vi "SeverNanonisSSL.vi"() -> ()   [LabVIEW 2014]
uses:
  <userlib>/SSL Library/Controls/SSL_Data.ctl
  <userlib>/SSL Library/Controls/Ref.ctl
  <userlib>/SSL Library/SSL Lib.lvlib
panel:
  out "Auth Status":T1(ring)
  in  "User":cluster{"pass":string, "User":string}={"pass"="password", "User"="password"}
  out "User auth":bool
  out "Listener Ref":refnum<k24>
  out "Client Connected ?":bool
  in  "Ssl Protocols Type":i32(ring)=240 items=["None"=0, "Ssl2"=12, "Ssl3"=48, "Tls"=192, "Default"=240]
  in  "Client Certificate Required":bool
  in  "Input Message":string="keep alive,30000;" caption="Type Message to send"
  out "Message log":string
  in  "Port Number":i32=4001
  out "Status":string="Waiting For Client ..."
  in  "Stop Button":bool=TRUE
  in  "Restart":bool
  in  "Read":bool
  in  "Write":bool
  out "Error Out":errorcluster
  in  "Password":string="password"
  in  "Certificate Path":string="C:\\Program Files (x86)\\National Instruments\\LabVIEW 2014\\user.lib\\SSL Library\\Server.pfx"
  in  "Error In":errorcluster
  # "TCP Server over SSL"
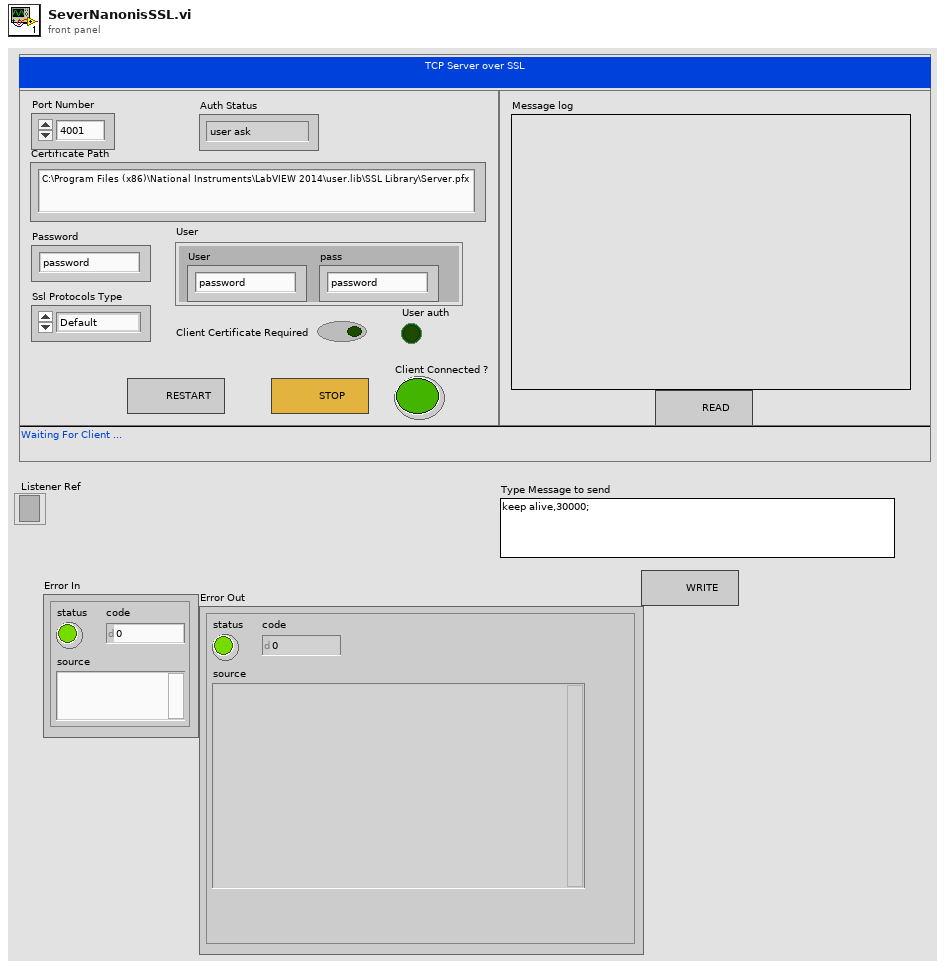
[diagram p1: front panel]
types:
  T1 = enum16{"user ask", "user", "pass ask", "pass", "auth"}
  T2 = typedef "SSL_Data.ctl" = cluster{"Listener Ref":refnum<k24>, "Certificate":refnum<k24>, "AcceptTcpClient":refnum<k24>, "SSL Stream":refnum<k24>, "Message Read":string}
  T3 = enum16{"Poll", "Open Listener", "Generate Certificate", "Wait for Client", "Open SSL Steram", "Read from SSL Stream", "Write Data to SSL Steram", "Close Connection"}
  T4 = typedef "Ref.ctl" = enum16{"Update Ref", "Read Ref", "Close Ref"}
  T5 = cluster{"Certificate Ref":refnum<k24>, "Client Certificate Required":bool, "Ssl Protocols Type":i32, "Check Certificate Revocation":bool}
  T6 = enum16{"Poll", "Open Listener", "Generate Certificate", "Wait for Client", "Open SSL Steram", "Read from SSL Stream", "Write Data to SSL Steram", "Close Connection", "Ask Username", "Ask Password", "Parse"}
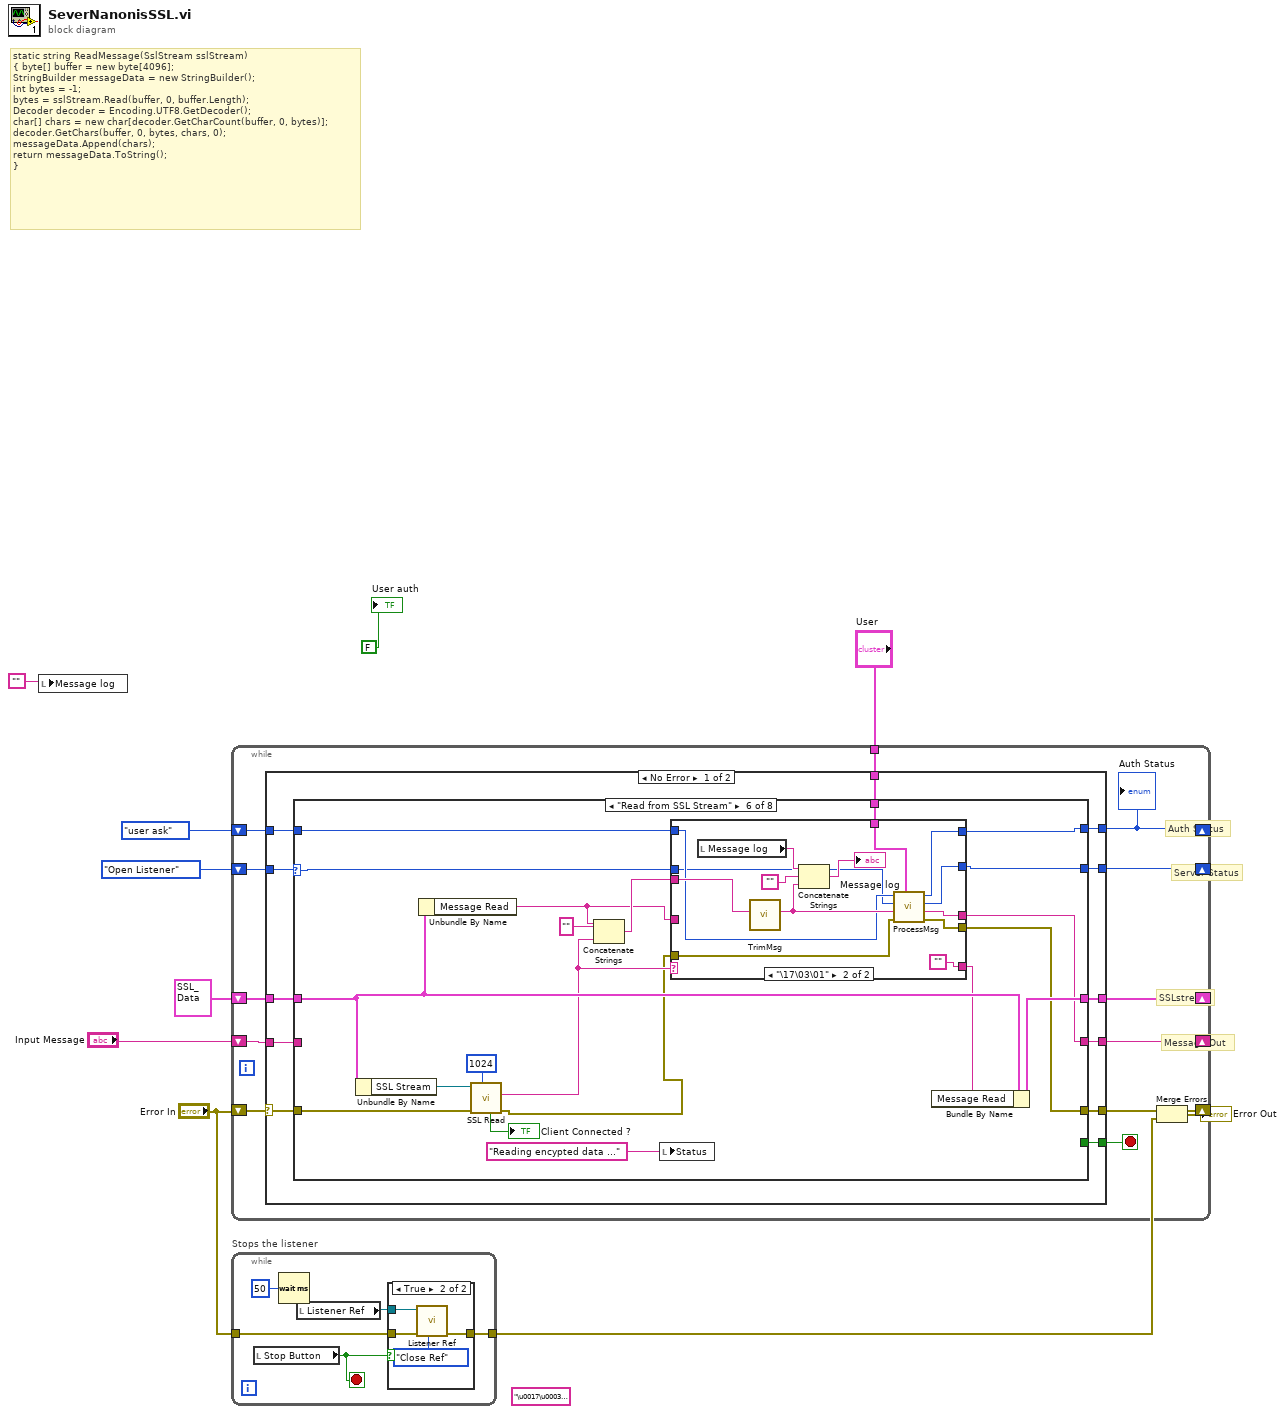
[diagram p0: block diagram]
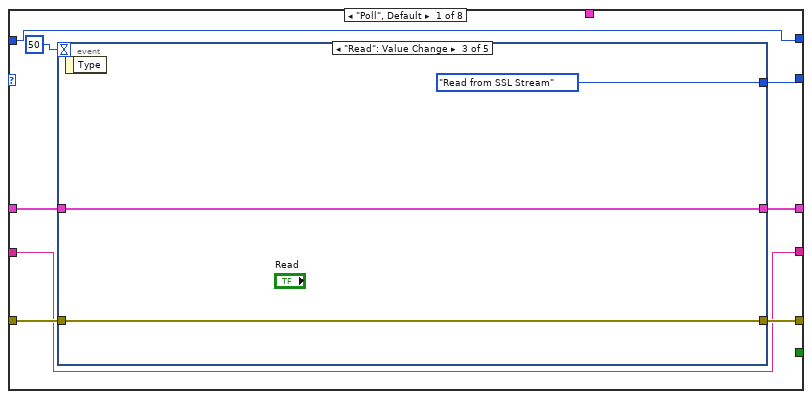
[diagram p3: hidden frame]
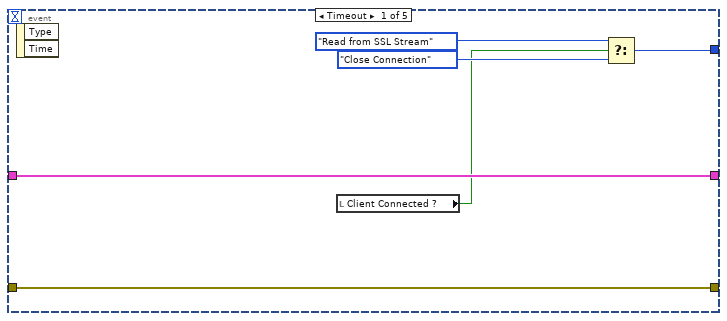
[diagram p4: hidden frame]
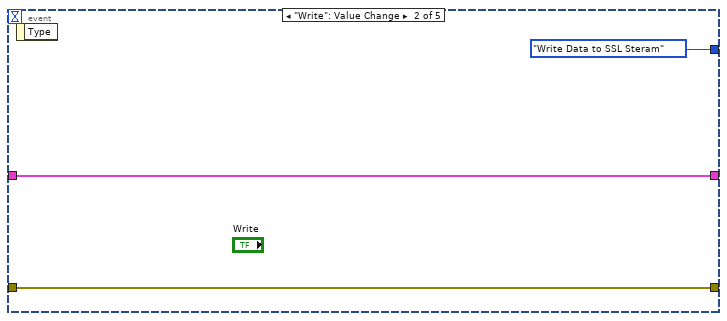
[diagram p5: hidden frame]
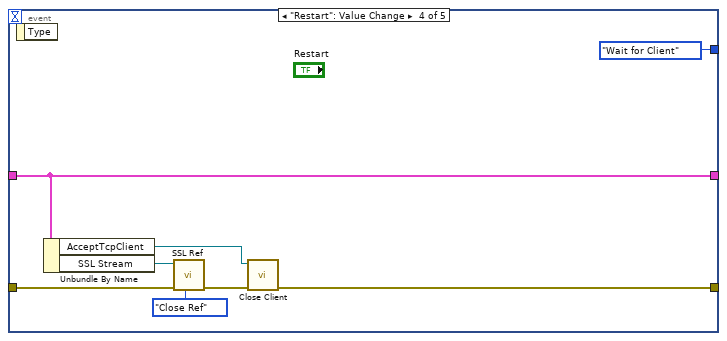
[diagram p6: hidden frame]
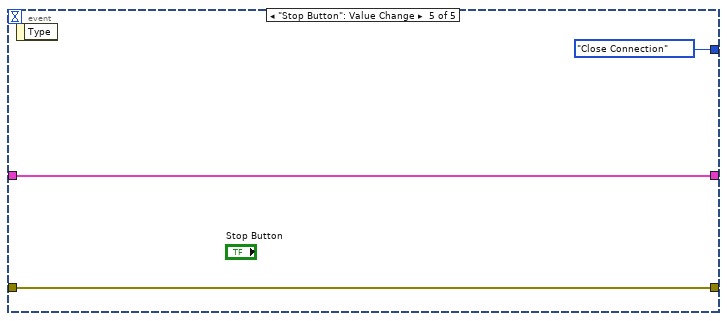
[diagram p7: hidden frame]
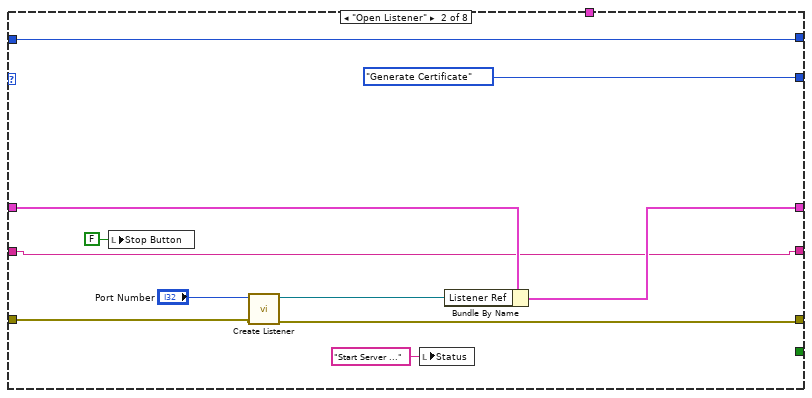
[diagram p8: hidden frame]
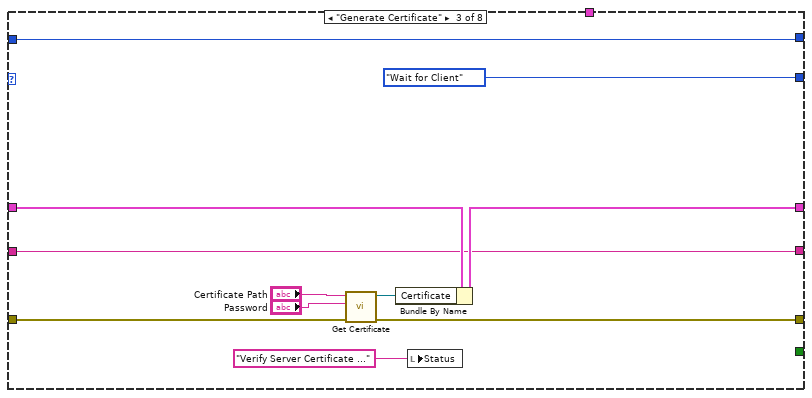
[diagram p9: hidden frame]
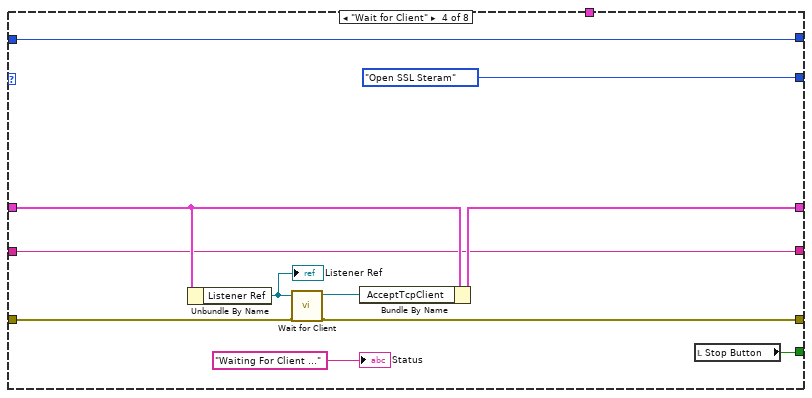
[diagram p10: hidden frame]
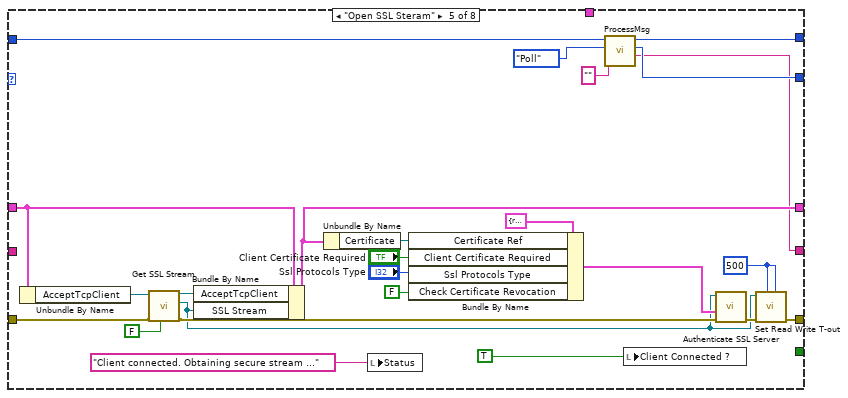
[diagram p11: hidden frame]
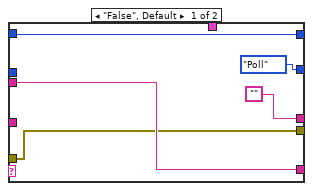
[diagram p12: hidden frame]
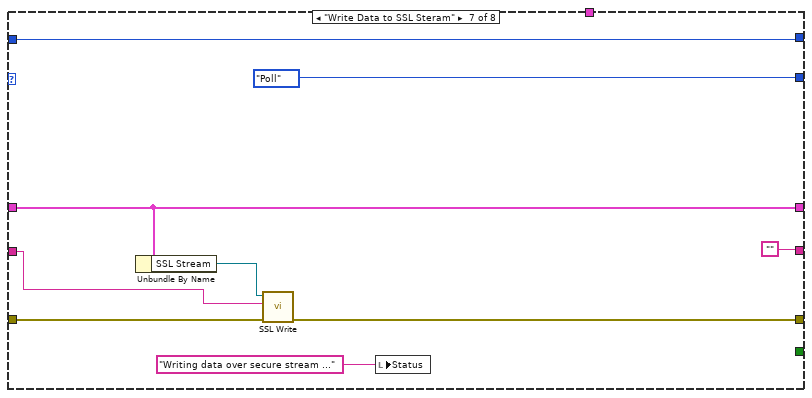
[diagram p13: hidden frame]
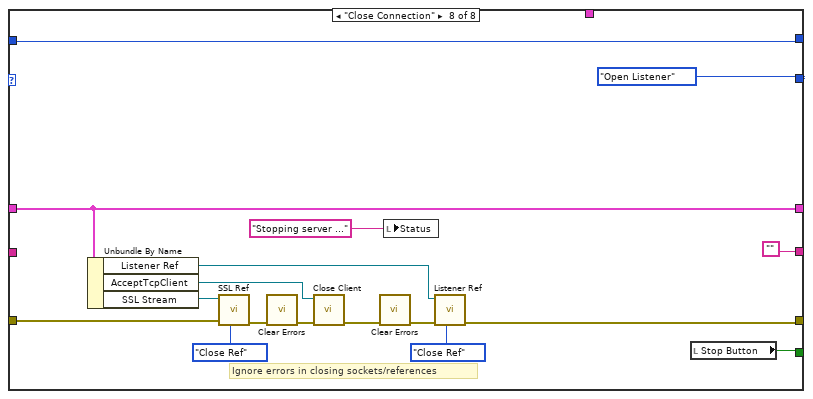
[diagram p14: hidden frame]
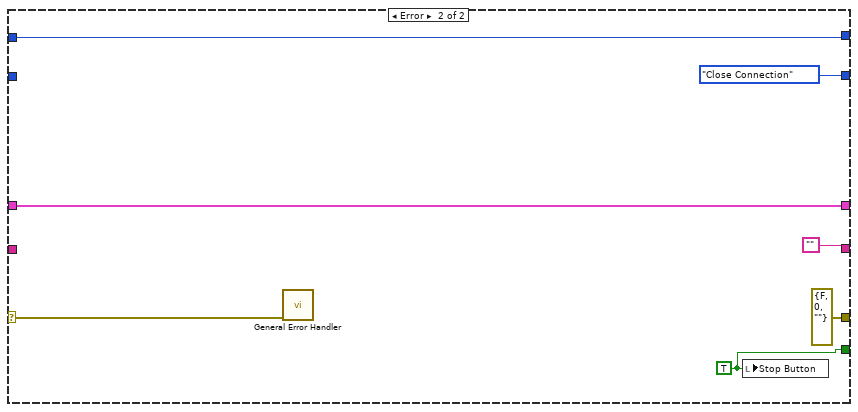
[diagram p15: hidden frame]
diagram:
  (unwired) "\u0017\u0003\u0001"
  # "Server Status"
  # "Auth Status"
  # "SSLstream"
  # "Message Out"
  # "static string ReadMessage(SslStream sslStream) \n{ byte[] buffer = new byte[4096];\nStringBuilder messageData = new StringBuilder(); \nint bytes = -1;\nbytes = sslStream.Read(buffer, 0, buffer.Length);\nDecoder decoder = Encoding.UTF8.GetDecoder(); \nchar[] chars = new char[decoder.GetCharCount(buffer, 0, bytes)]; \ndecoder.GetChars(buffer, 0, bytes, chars, 0); \nmessageData.Append(chars);\nreturn messageData.ToString();\n}"
  n1 = local write "Message log"("") -> ()
  n2 = while {
    shift-right: [w21] -> _
    shift-left: T2 {"Listener Ref"=refnum, "Certificate"=refnum, "AcceptTcpClient"=refnum, "SSL Stream"=refnum, "Message Read"=""} -> [w22]
    shift-right: [w23] -> w8
    shift-left: "Error In" -> [w20]
    shift-right: [w18] -> _
    shift-left: T3."Open Listener" -> [w19]
    shift-right: [w15] -> _
    shift-left: T1."user ask" -> [w16]
    shift-right: [w13] -> _
    shift-left: "Input Message" -> [w14]
    tunnel: "User" -> [w12]
    stop <- w17 stop-if-true
    n3 = case shown="No Error" w20 {
      selector: w20 -> [w32 w194]
      tunnel: [w35 errorcluster {"status"=FALSE, "code"=0, "source"=""} ("Error Out")] -> w23
      tunnel: w22 -> [w34 w196]
      tunnel: [w33 w196] -> w21
      tunnel: w19 -> [w31 _]
      tunnel: [w30 T3."Close Connection"] -> w18
      tunnel: [w29 w192] -> w17
      tunnel: w16 -> [w28 w191]
      tunnel: [w27 w191] -> w15
      tunnel: w14 -> [w26 _]
      tunnel: [w25 ""] -> w13
      tunnel: w12 -> [w24 _]
      frame No Error {
        n4 = case shown="\"Read from SSL Stream\"" w31 {
          selector: w31 -> [_ _ _ _ _ w130 _ _]
          tunnel: w32 -> [w41 w76 w85 w96 w124 w144 w171 w188]
          tunnel: [w40 w75 w84 w95 w109 w126 w170 w184] -> w35
          tunnel: w34 -> [w43 w70 w88 w93 w121 w140 w168 w179]
          tunnel: [w42 w69 w87 w99 w117 w139 w168 w179] -> w33
          tunnel: [w39 T3."Generate Certificate" T3."Wait for Client" T3."Open SSL Steram" w102 w129 T3."Poll" T3."Open Listener"] -> w30
          tunnel: [_ _ _ w89 _ _ _ w173] -> w29
          tunnel: w28 -> [w37 w68 w79 w91 w105 w132 w166 w174]
          tunnel: [w37 w68 w79 w91 w104 w131 w166 w174] -> w27
          tunnel: w26 -> [w36 w67 w78 w90 _ _ w165 _]
          tunnel: [w36 w67 w78 w90 w100 w128 "" ""] -> w25
          tunnel: w24 -> [_ _ _ _ _ w125 _ _]
          frame "Poll", Default {
            n5 = event shown="[2] \"Read\": Value Change" {
              selector: _ -> [_ _ _ _ _]
              dyn-events: _ -> [_ _ _ _ _]
              timeout: 50 -> [_ _ _ _ _]
              tunnel: w43 -> [w46 w52 w55 w58 w65]
              tunnel: [w46 w52 w55 w58 w65] -> w42
              tunnel: w41 -> [w45 w51 w54 w62 w66]
              tunnel: [w45 w51 w54 w60 w66] -> w40
              tunnel: [w49 T3."Write Data to SSL Steram" T3."Read from SSL Stream" T3."Wait for Client" T3."Close Connection"] -> w39
              event Timeout {
                n6 = event-data() -> ()  [unwired: 1 in, 2 out]
                n7 = local read "Client Connected ?"() -> (w44:bool)
                n8 = Select(t=T3."Read from SSL Stream", s=w44, f=T3."Close Connection") -> (s? t:f=w49:T3)
              }
              event "Write": Value Change {
                n9 = event-data() -> ()  [unwired: 1 in, 1 out]
              }
              event "Read": Value Change {
                n10 = event-data() -> ()  [unwired: 1 in, 1 out]
              }
              event "Restart": Value Change {
                n11 = event-data() -> ()  [unwired: 1 in, 1 out]
                n12 = Unbundle By Name(w58) -> ("AcceptTcpClient"=w56:refnum<k24>, "SSL Stream"=w57:refnum<k24>)
                n13 = call <userlib>:"SSL Ref.vi"("Action"=Ref."Close Ref", "Error In"=w62, "SSL Stream"=w57) -> ("Error Out"=w61:errorcluster)  [unwired: 7 in, 1 out]
                n14 = call <userlib>:"Close Client.vi"("Error In"=w61, "Client Ref"=w56) -> ("Error Out"=w60:errorcluster)  [unwired: 9 in]
              }
              event "Stop Button": Value Change {
                n15 = event-data() -> ()  [unwired: 1 in, 1 out]
              }
            }
          }
          frame "Open Listener" {
            n16 = local write "Stop Button"(FALSE ("Stop Button")) -> ()
            n17 = call <userlib>:"Create Listener.vi"("Error In"=w76, "Port Number"="Port Number") -> ("Error Out"=w75:errorcluster, "Listener"=w71:refnum<k24>)  [unwired: 8 in]
            n18 = local write "Status"("Start Server ..." ("Status")) -> ()
            n19 = Bundle By Name(cluster=w70, "Listener Ref"=w71) -> (w69:T2)
          }
          frame "Generate Certificate" {
            n20 = call <userlib>:"Get Certificate.vi"("Error In"=w85, "Password"="Password", "Certificate Path"="Certificate Path") -> ("Error Out"=w84:errorcluster, "Certificate"=w83:refnum<k24>)  [unwired: 6 in, 1 out]
            n21 = Bundle By Name(cluster=w88, "Certificate"=w83) -> (w87:T2)
            n22 = local write "Status"("Verify Server Certificate ..." ("Status")) -> ()
          }
          frame "Wait for Client" {
            n23 = Unbundle By Name(w93) -> ("Listener Ref"=w92:refnum<k24>)
            "Listener Ref" <- w92
            n24 = call <userlib>:"Wait for Client.vi"("Error In"=w96, "Listener Ref"=w92) -> ("Error Out"=w95:errorcluster, "Client Ref"=w94:refnum<k24>)  [unwired: 8 in]
            n25 = Bundle By Name(cluster=w93, "AcceptTcpClient"=w94) -> (w99:T2)
            n26 = local read "Stop Button"() -> (w89:bool)
            "Status" <- "Waiting For Client ..." ("Status")
          }
          frame "Open SSL Steram" {
            w107 = 500 ("Read Timeout(in ms)")
            n27 = Unbundle By Name(w121) -> ("AcceptTcpClient"=w122:refnum<k24>)
            n28 = call <userlib>:"Get SSL Stream.vi"("Leave Inner Stream Open"=FALSE, "Error In"=w124, "Client Ref"=w122) -> ("Error Out"=w119:errorcluster, "SSL Ref"=w108:refnum<k24>, "Client Ref"=w120:refnum<k24>)  [unwired: 6 in]
            n29 = Bundle By Name(cluster=w121, "AcceptTcpClient"=w120, "SSL Stream"=w108) -> (w117:T2)
            n30 = Unbundle By Name(w117) -> ("Certificate"=w116:refnum<k24>)
            n31 = local write "Status"("Client connected. Obtaining secure stream ..." ("Status")) -> ()
            n32 = Bundle By Name(cluster=T5 {"Certificate Ref"=refnum, "Client Certificate Required"=FALSE, "Ssl Protocols Type"=0, "Check Certificate Revocation"=FALSE} ("Input Data"), "Certificate Ref"=w116, "Client Certificate Required"="Client Certificate Required", "Ssl Protocols Type"="Ssl Protocols Type", "Check Certificate Revocation"=FALSE) -> (w115:T5)
            n33 = call <userlib>:"ProcessMsg.vi"("MessageIn"="", "ServerStatus"=T3."Poll", "Auth Status"=w105) -> ("MessageOut"=w100:string, "ServerStatus out"=w102:T6, "Auth Status Out"=w104:T1)  [unwired: 5 in, 1 out]
            n34 = local write "Client Connected ?"(TRUE ("Client Connected ?")) -> ()
            n35 = call <userlib>:"Authenticate SSL Server.vi"("Error In"=w119, "Input Data"=w115, "SSL Stream"=w108) -> ("Error Out"=w110:errorcluster)  [unwired: 8 in]
            n36 = call <userlib>:"Set Read Write T-out.vi"("Write Timeout(in ms)"=w107, "Read Timeout(in ms)"=w107, "Error In"=w110, "SSL Stream"=w108) -> ("Error Out"=w109:errorcluster)  [unwired: 7 in]
          }
          frame "Read from SSL Stream" {
            n37 = Unbundle By Name(w140) -> ("SSL Stream"=w141:refnum<k24>)
            n38 = Unbundle By Name(w140) -> ("Message Read"=w134:string)
            n39 = call <userlib>:"SSL Read.vi"("Buffer Size"=1024, "Error In"=w144, "SSL Stream"=w141) -> ("Error Out"=w127:errorcluster, "Message Read"=w135:string, "Client Connected ?"=→"Client Connected ?":bool)  [unwired: 6 in]
            n40 = Concatenate Strings(w134, "" ("string"), w135) -> (w137:string)
            n41 = local write "Status"("Reading encypted data ..." ("Status")) -> ()
            n42 = case shown="\"\\17\\03\\01\"" w135 {
              tunnel: w134 -> [_ _]
              tunnel: [w149 ""] -> w138
              tunnel: w137 -> [w149 w163]
              tunnel: w132 -> [w146 w159]
              tunnel: [w146 w158] -> w131
              tunnel: w130 -> [_ w157]
              tunnel: [T3."Poll" w156] -> w129
              tunnel: ["" w155] -> w128
              tunnel: w127 -> [w145 w154]
              tunnel: [w145 w153] -> w126
              tunnel: w125 -> [_ w150]
              frame "False", Default {
              }
              frame "\u0017\u0003\u0001" {
                n43 = local read "Message log"() -> (w162:string)
                n44 = call <userlib>:"TrimMsg.vi"("Message"=w163) -> ("Msg"=w160:string)  [unwired: 10 in]
                n45 = Concatenate Strings(w162, "", w160) -> (→"Message log":string)
                n46 = call <userlib>:"ProcessMsg.vi"("User"=w150, "Error In"=w154, "MessageIn"=w160, "ServerStatus"=w157, "Auth Status"=w159) -> ("Error Out"=w153:errorcluster, "MessageOut"=w155:string, "ServerStatus out"=w156:T6, "Auth Status Out"=w158:T1)  [unwired: 3 in]
              }
            }
            n47 = Bundle By Name(cluster=w140, "Message Read"=w138) -> (w139:T2)
          }
          frame "Write Data to SSL Steram" {
            n48 = Unbundle By Name(w168) -> ("SSL Stream"=w167:refnum<k24>)
            n49 = call <userlib>:"SSL Write.vi"("Error In"=w171, "Input Message"=w165, "SSL Stream"=w167) -> ("Error Out"=w170:errorcluster)  [unwired: 8 in]
            n50 = local write "Status"("Writing data over secure stream ..." ("Status")) -> ()
          }
          frame "Close Connection" {
            # "Ignore errors in closing sockets/references"
            n51 = Unbundle By Name(w179) -> ("Listener Ref"=w176:refnum<k24>, "AcceptTcpClient"=w177:refnum<k24>, "SSL Stream"=w178:refnum<k24>)
            n52 = call <userlib>:"SSL Ref.vi"("Action"=Ref."Close Ref", "Error In"=w188, "SSL Stream"=w178) -> ("Error Out"=w187:errorcluster)  [unwired: 7 in, 1 out]
            n53 = call <vilib>:"Clear Errors.vi"("error in (no error)"=w187) -> ("error out"=w181:errorcluster)  [unwired: 5 in, 1 out]
            n54 = call <userlib>:"Close Client.vi"("Error In"=w181, "Client Ref"=w177) -> ("Error Out"=w185:errorcluster)  [unwired: 9 in]
            n55 = call <vilib>:"Clear Errors.vi"("error in (no error)"=w185) -> ("error out"=w180:errorcluster)  [unwired: 5 in, 1 out]
            n56 = local write "Status"("Stopping server ..." ("Status")) -> ()
            n57 = call <userlib>:"Listener Ref.vi"("Action"=Ref."Close Ref", "Error In"=w180, "Listener Ref"=w176) -> ("Error Out"=w184:errorcluster)  [unwired: 7 in, 1 out]
            n58 = local read "Stop Button"() -> (w173:bool)
          }
        }
      }
      frame Error {
        w192 = TRUE
        n59 = call <vilib>:"General Error Handler.vi"("error in (no error)"=w194) -> ()  [unwired: 10 in, 5 out]
        n60 = local write "Stop Button"(w192) -> ()
      }
    }
    "Auth Status" <- w15
  }
  n61 = while "Stops the listener" {
    tunnel: "Error In" -> [w200]
    tunnel: [w198] -> w7
    stop <- w201 stop-if-true
    n62 = local read "Stop Button"() -> (w201:bool)
    n63 = Wait (ms)(milliseconds to wait=u32 50) -> ()  [unwired: 1 out]
    n64 = local read "Listener Ref"() -> (w197:refnum<k24>)
    n65 = case shown="True" w201 {
      tunnel: w200 -> [w202 w205]
      tunnel: [w202 w204] -> w198
      tunnel: w197 -> [_ w203]
      frame False {
      }
      frame True {
        n66 = call <userlib>:"Listener Ref.vi"("Action"=Ref."Close Ref", "Error In"=w205, "Listener Ref"=w203) -> ("Error Out"=w204:errorcluster)  [unwired: 7 in, 1 out]
      }
    }
  }
  n67 = Merge Errors(w8, w7) -> (→"Error Out":errorcluster)
  "User auth" <- FALSE ("User auth")
